vi "_FPGA_DDS_CrossZeroPhase.vi"(1 "RfCyc_in":u64) -> (0 "Cross Zero Phase?":bool)   [LabVIEW 2018]
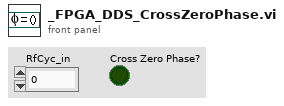
[diagram p1: front panel]
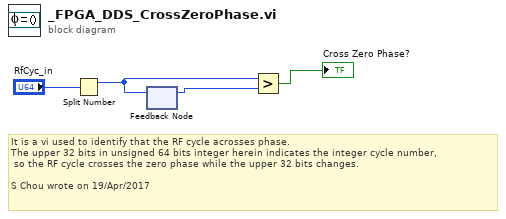
[diagram p0: block diagram]
diagram:
  # "It is a vi used to identify that the RF cycle acrosses phase.\nThe upper 32 bits in unsigned 64 bits integer herein indicates the integer cycle number,\n so the RF cycle crosses the zero phase while the upper 32 bits changes.\n\nS Chou wrote on 19/Apr/2017"
  n1 = Split Number(x="RfCyc_in") -> (hi(x)=w3:u32)  [unwired: 1 out]
  n2 = feedback #1() -> (w1:u32)  [unwired: 1 in]
  n3 = feedback-in #1(w3) -> ()
  n4 = Greater?(x=w3, y=w1) -> (0:→"Cross Zero Phase?":bool)
